vi "Cleanup Client If Error.vi"(8 "error in":errorcluster, 10 "client name":string, 11 "project ref in":refnum<vi>) -> (0 "error out":errorcluster, 1 "status":T1, 2 "error message":string, 3 "project ref out":refnum<vi>)   [LabVIEW 2021, in "MeasurementClient Editor.lvlib"]
uses:
  MeasurementClient Editor.lvlib
  Client Creation Status.ctl
  <vilib>/Utility/error.llb/DialogType.ctl
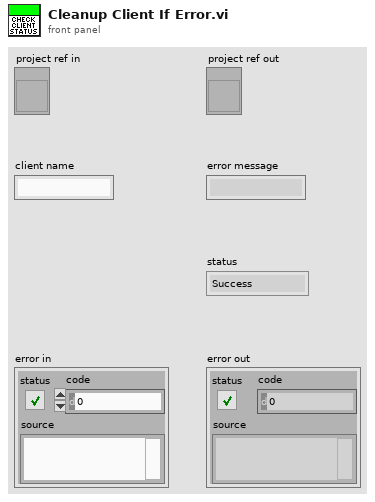
[diagram p1: front panel]
types:
  T1 = typedef "MeasurementClient Editor.lvlib/Client Creation Status.ctl" = enum16{"Success", "Fail"}
  T2 = typedef "DialogType.ctl" = u16
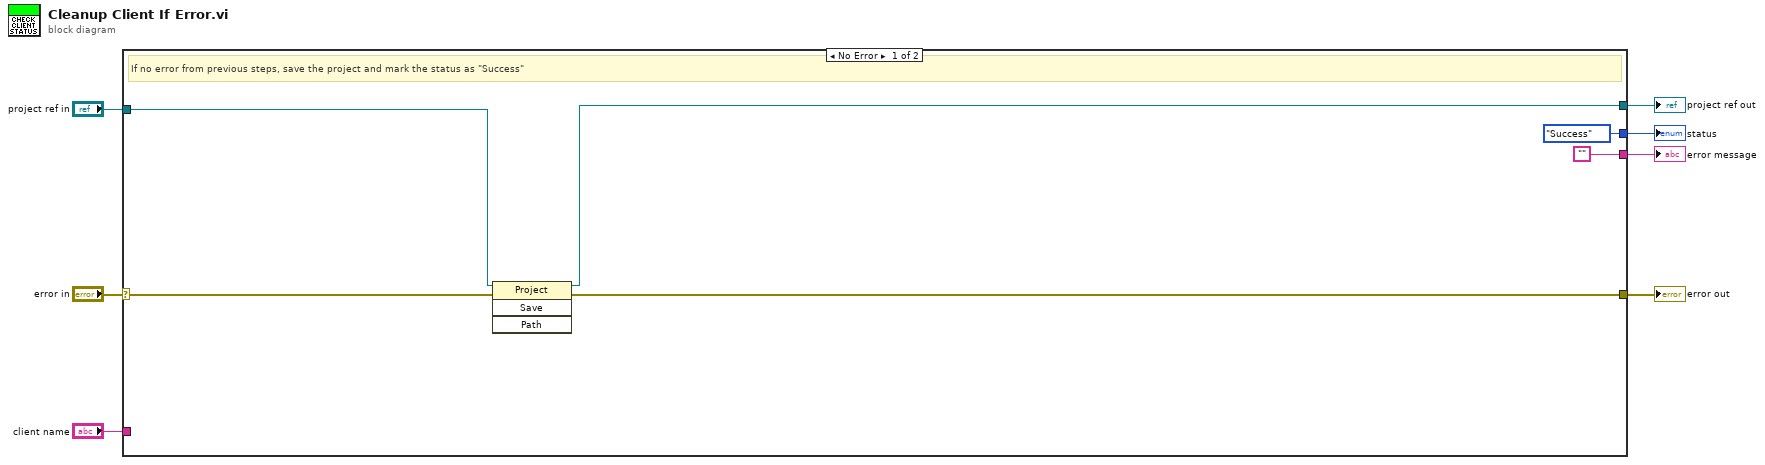
[diagram p0: block diagram]
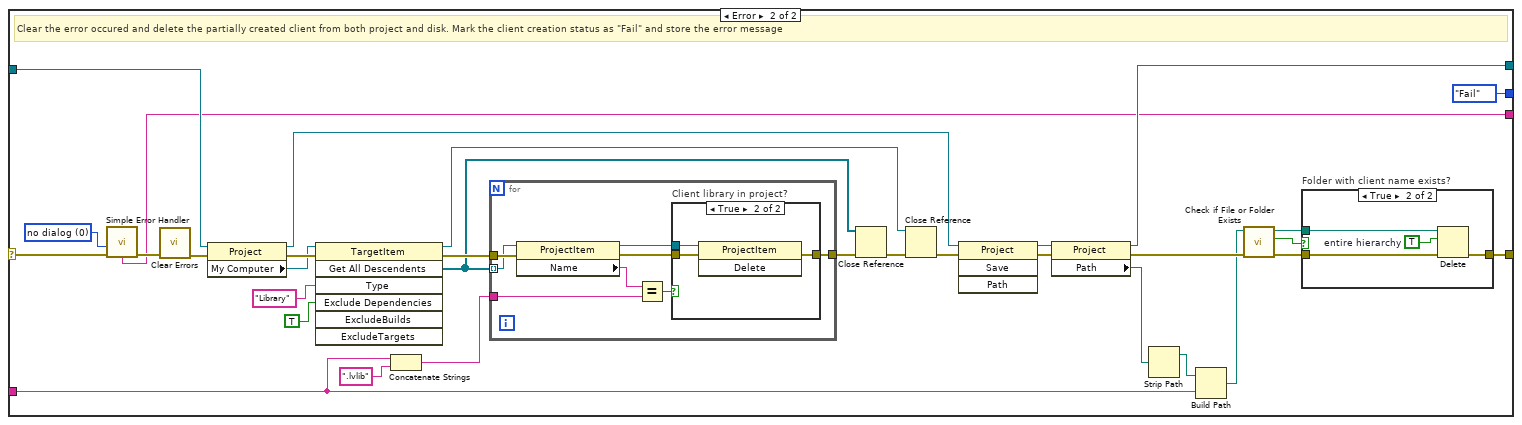
[diagram p2: hidden frame]
diagram:
  n1 = case shown="No Error" "error in" {
    selector: "error in" -> [w13 w37]
    tunnel: [w10 w28] -> w7
    tunnel: "project ref in" -> [w12 w45]
    tunnel: [w11 w33] -> w4
    tunnel: [Client_Creation_Status."Success" Client_Creation_Status."Fail"] -> w1
    tunnel: ["" w17] -> w3
    tunnel: "client name" -> [_ w22]
    frame No Error {
      # "If no error from previous steps, save the project and mark the status as \"Success\""
      n2 = invoke class="Project" method="Save"(reference=w12, error in=w13) -> (reference out=w11:refnum<vi>, error out=w10:errorcluster)  [unwired: 2 in, 2 out]
    }
    frame Error {
      w18 = T2 0 items=["no dialog", "OK message", "continue or stop message", "OK message + warnings", "continue/stop + warnings"] ("type of dialog (OK msg:1)")
      # "Clear the error occured and delete the partially created client from both project and disk. Mark the client creation status as \"Fail\" and store the error message"
      n3 = call <vilib>:"Simple Error Handler.vi"("type of dialog (OK msg:1)"=w18, "error in (no error)"=w37) -> ("error out"=w19:errorcluster, "message"=w17:string)  [unwired: 3 in, 3 out]
      n4 = call <vilib>:"Clear Errors.vi"("error in (no error)"=w19) -> ("error out"=w38:errorcluster)  [unwired: 5 in, 1 out]
      n5 = property class="Project"(reference=w45, error in=w38) -> (reference out=w25:refnum<vi>, error out=w44:errorcluster, "My Computer"=w43:refnum<vi>)
      n6 = invoke class="TargetItem" method="Get All Descendents"(reference=w43, error in=w44, "Type"="Library", "Exclude Dependencies"=TRUE ("ExcludeDependencies")) -> (reference out=w35:refnum<vi>, error out=w40:errorcluster, "All Descendents"=w15:refnum<vi>[])  [unwired: 3 in, 4 out]
      n7 = Concatenate Strings(w22, ".lvlib" ("string")) -> (w21:string)
      n8 = for {
        tunnel: w40 -> [w58]
        tunnel: w15 -> [w57] mode=indexing
        tunnel: w21 -> [w55]
        tunnel: [w51] -> w39
        n9 = property class="ProjectItem"(reference=w57, error in=w58) -> (reference out=w54:refnum<vi>, error out=w52:errorcluster, "Name"=w56:string)
        n10 = Equal?(x=w56, y=w55) -> (x = y?=w53:bool)
        n11 = case "Client library in project?" shown="True" w53 {
          tunnel: w54 -> [_ w62]
          tunnel: w52 -> [w59 w61]
          tunnel: [w59 w60] -> w51
          frame False {
          }
          frame True {
            n12 = invoke class="ProjectItem" method="Delete"(reference=w62, error in=w61) -> (error out=w60:errorcluster)  [unwired: 1 in, 2 out]
          }
        }
      }
      n13 = Close Reference(reference=w15, error in (no error)=w39) -> (error out=w16:errorcluster)
      n14 = Close Reference(reference=w35, error in (no error)=w16) -> (error out=w36:errorcluster)
      n15 = invoke class="Project" method="Save"(reference=w25, error in=w36) -> (reference out=w24:refnum<vi>, error out=w26:errorcluster)  [unwired: 2 in, 2 out]
      n16 = property class="Project"(reference=w24, error in=w26) -> (reference out=w33:refnum<vi>, error out=w34:errorcluster, "Path"=w32:path)
      n17 = Strip Path(path=w32) -> (stripped path=w31:path)  [unwired: 1 out]
      n18 = Build Path(base path=w31, name or relative path=w22) -> (appended path=w30:path)
      n19 = call <vilib>:"Check if File or Folder Exists.vi"("error in (no error)"=w34, "path"=w30) -> ("error out"=w29:errorcluster, "file or folder exists?"=w20:bool, "dup path"=w27:path)  [unwired: 7 in]
      n20 = case "Folder with client name exists?" shown="True" w20 {
        tunnel: w29 -> [w46 w50]
        tunnel: [w46 w49] -> w28
        tunnel: w27 -> [_ w48]
        frame False {
        }
        frame True {
          w47 = TRUE  # entire hierarchy
          n21 = Delete(path (use dialog)=w48, entire hierarchy (F)=w47, error in=w50) -> (error out=w49:errorcluster)  [unwired: 2 in, 2 out]
        }
      }
    }
  }
  "project ref out" <- w4
  "error out" <- w7
  "error message" <- w3
  "status" <- w1
